vi "Trig Rate Charactarization.vi"(7 "Reset latch":refnum<vi>, 8 "error in (no error)":errorcluster, 9 "Programmatic set Vtrig":refnum<vi>, 11 "VTrig mV":refnum<vi>) -> (0 "Error out":errorcluster)   [LabVIEW 2016]
uses:
  <vilib>/Platform/TimedLoop/XDataNode/timing_clust.ctl
  <vilib>/Platform/TimedLoop/XDataNode/nitl_modes.ctl
  <vilib>/Platform/TimedLoop/XDataNode/wakeup.ctl
  <vilib>/platform/TimedLoop/XDataNode/XDataNode.xnode
  <vilib>/Platform/TimedLoop/XDataNode/XDNodeRunTimeDep.lvlib
  <vilib>/Analysis/NI_AALBase.lvlib
panel:
  out "Previous trigger level":dbl
  out "Trigger level increment":dbl
  out "Datapoints":i32
  out "Level number":i32
  out "Current\n trigger level":dbl
  in  "Datapoints per level":i32
  in  "finish level":bool
  in  "Bias being autoset?":bool=TRUE
  in  "MPPC Overvoltage":dbl
  in  "ROB ID":i32
  in  "MPPC Serial number":i32
  in  "Scintillator ID":i32
  in  "Data":i32[](array[numeric])
  out "Command Queue":string[](array[string])
  in  "stop":bool
  out "Hitrate histogram":T1(graph)
  out "Waveform Chart":dbl(graph)
  in  "Datasave path":path=path "D:/Data/Characterizations/Trigger rate characterizations"
  in  "Levels":i32
  in  "Range min":i32 format="%.0f  mV"
  in  "Range max":i32 format="%.0f mV"
  in  "Begin characterization":bool
  in  "Period":i32=1000 format="%.0f ms"
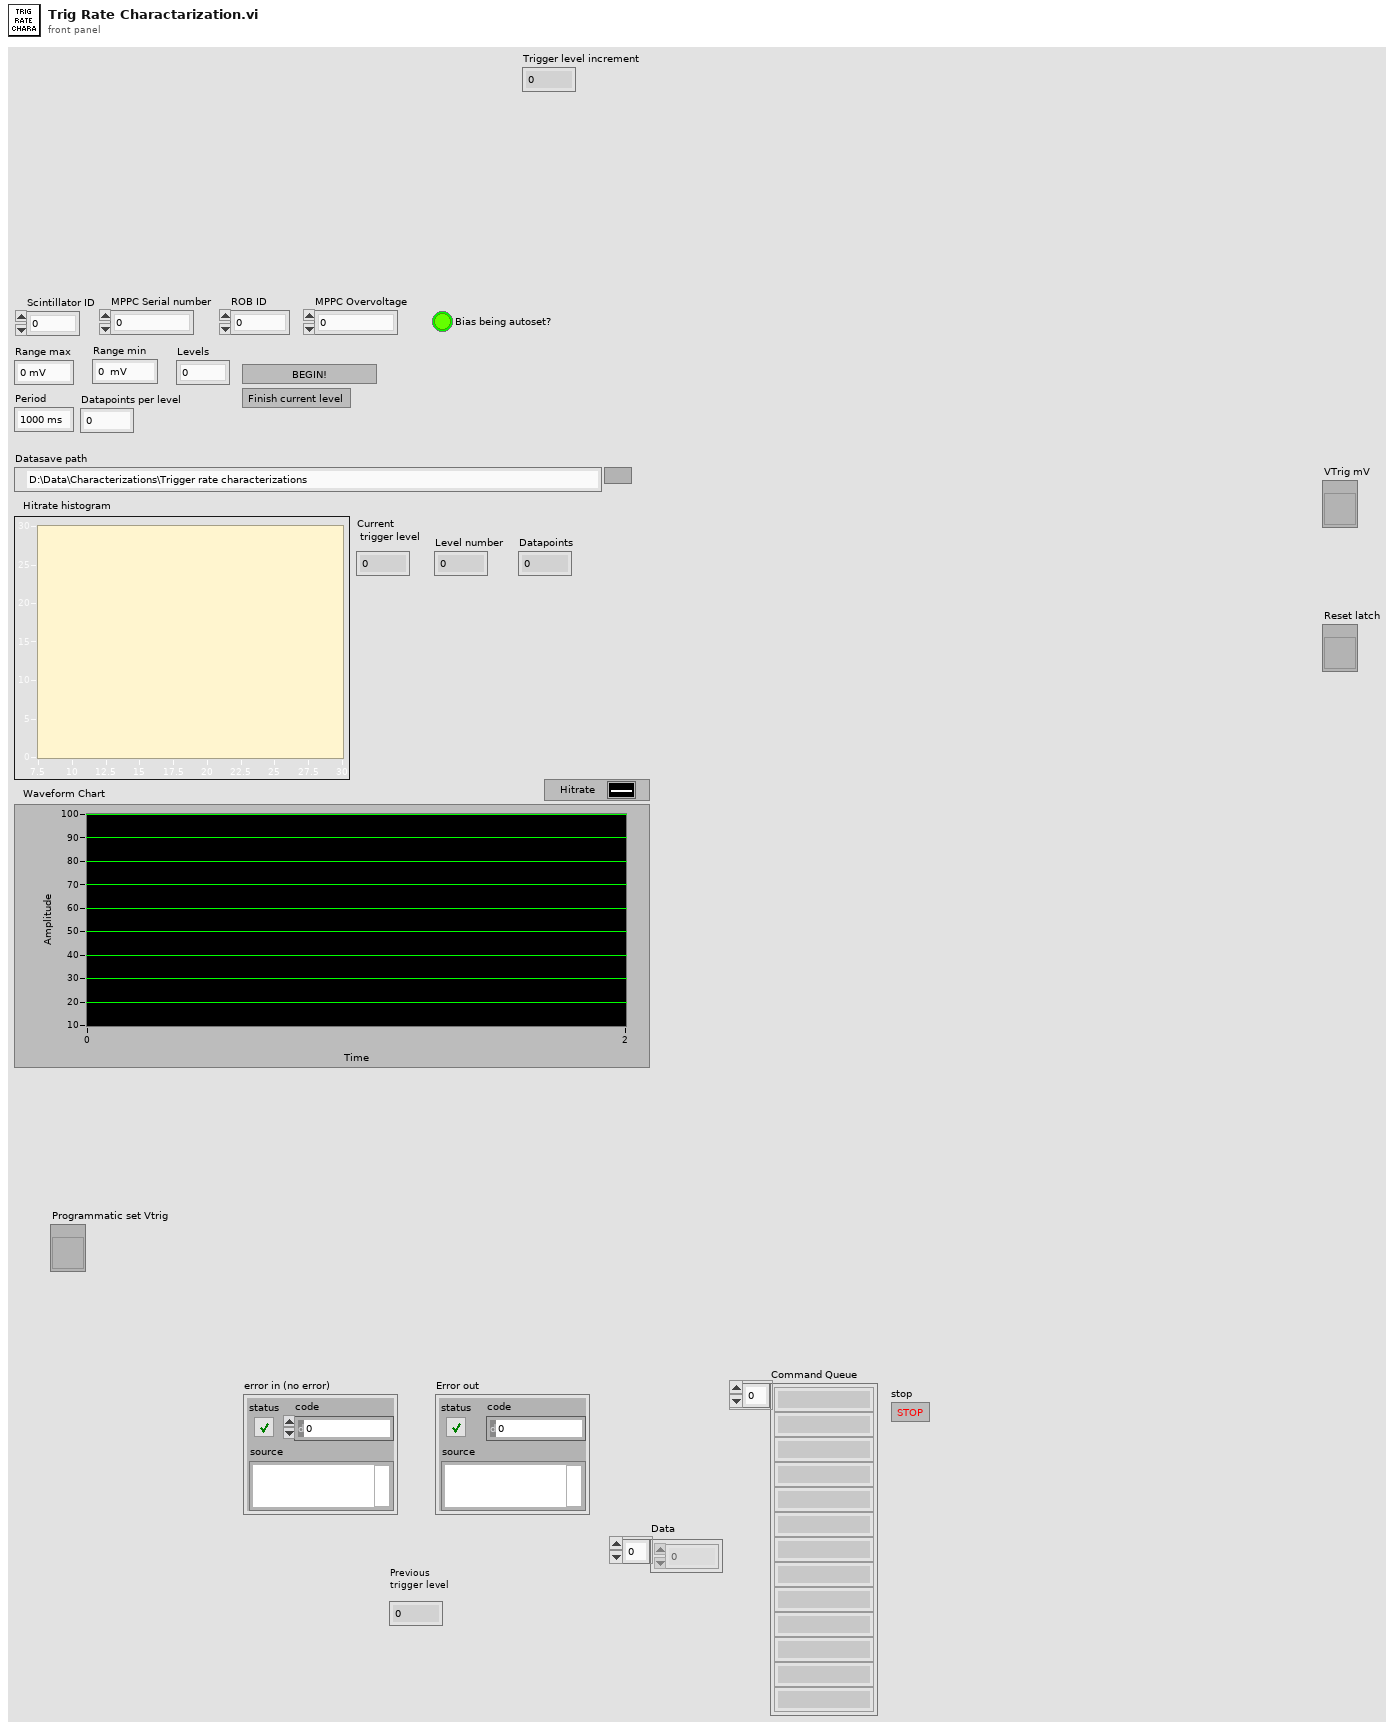
[diagram p1: front panel]
types:
  T1 = cluster{"X Values":dbl[], "Histogram: h(x)":i32[]}
  T2 = enum16{"open", "replace", "create", "open or create", "replace or create", "replace or create with confirmation"}
  T3 = enum16{"Reset", "ReadAndReset", "Read", "Add", "Init"}
  T4 = typedef "XDNodeRunTimeDep.lvlib/timing_clust.ctl" = cluster{"Expected End [f-1]":u64, "Actual End [f-1]":u64, "Finished Late? [f-1]":bool, "Expected End [i-1]":u64, "Actual End [i-1]":u64, "Finished Late? [i-1]":bool, "Expected Start [i]":u64, "Actual Start [i]":u64, "Expected Start [f]":u64, "Actual Start [f]":u64, "Source Name":string, "Structure Name":string, "Period":i64, "Deadline":i64, "Offset":i64, "Start":i64, "Priority":i32, "Timeout":i32, "Mode":T5, "Wakeup Reason":T6, "Error":errorcluster, "Source Type":string, "Secondary Source Type":string, "Global End Time":u64, "Global Start Time":u64, "Frame Duration":u64, "Iteration Duration":u64, "Assigned CPU":i32, "I/O Scan Engine Mode":u32}
  T5 = typedef "XDNodeRunTimeDep.lvlib/nitl_modes.ctl" = enum32{"No Change", "Process missed periods, maintain original phase", "Discard missed periods, maintain original phase", "Process missed periods, ignore original phase", "Discard missed periods, ignore original phase"}
  T6 = typedef "XDNodeRunTimeDep.lvlib/wakeup.ctl" = enum32{"Normal", "Aborted", "Asynchronous wakeup", "Timing source error", "Timed loop error", "Timeout"}
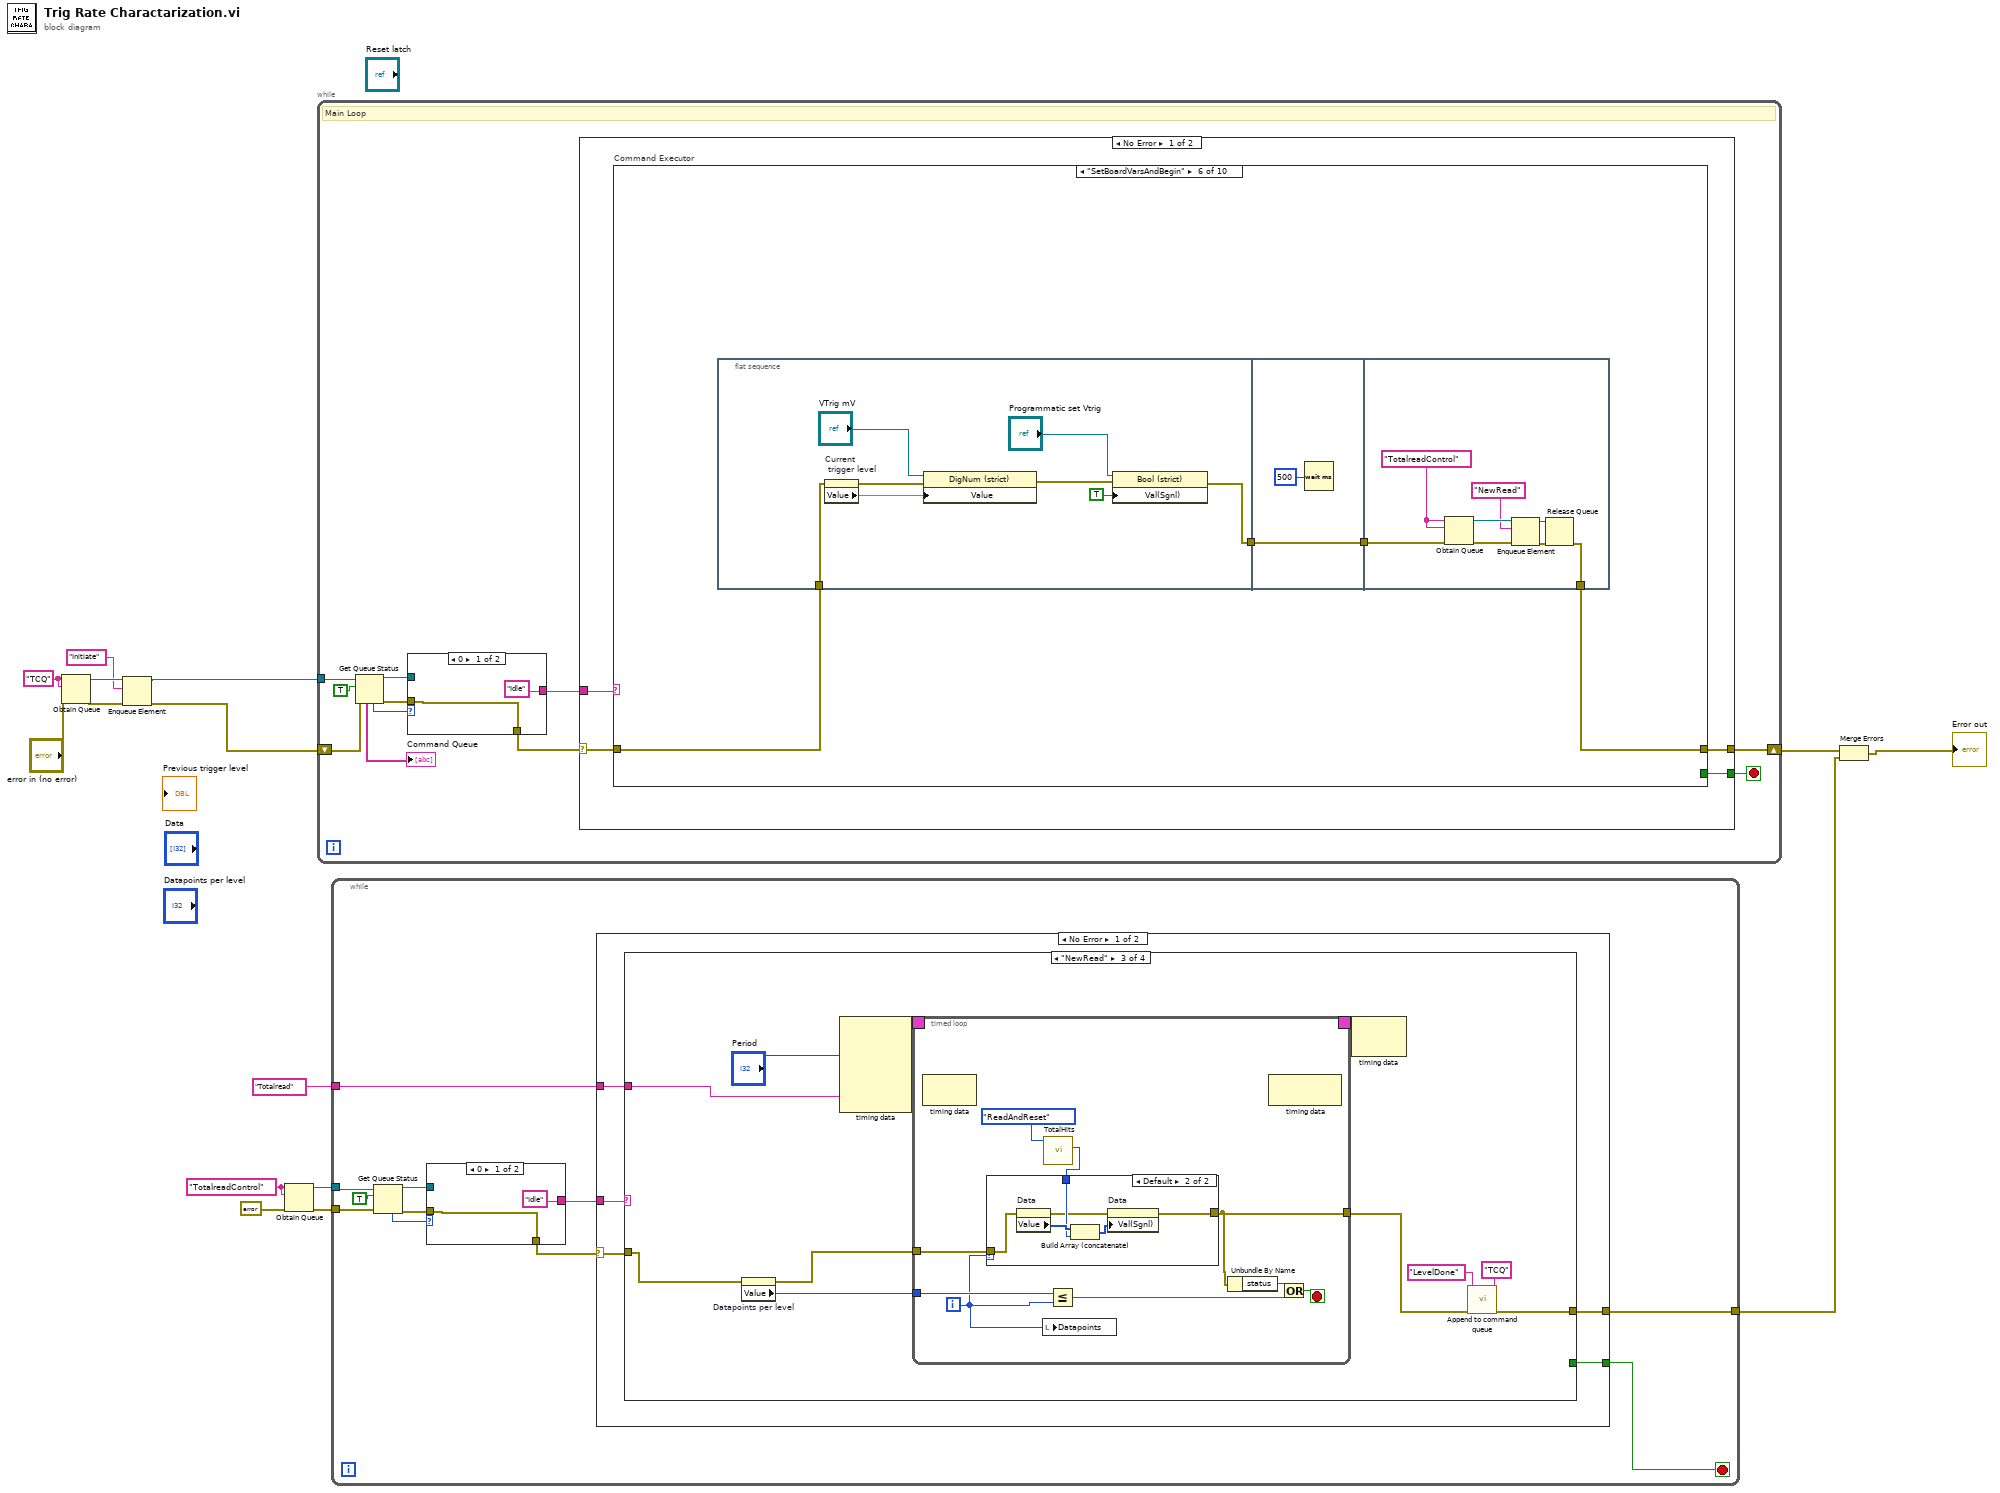
[diagram p0: block diagram]
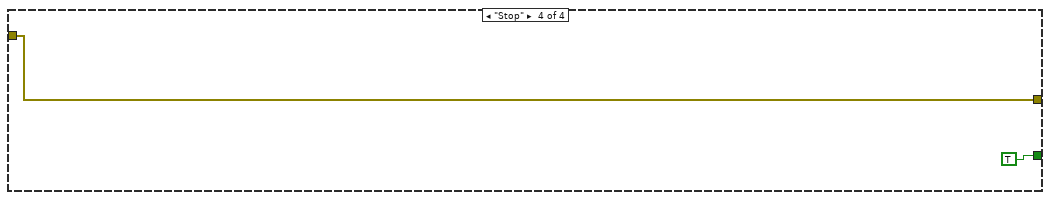
[diagram p5: hidden frame]
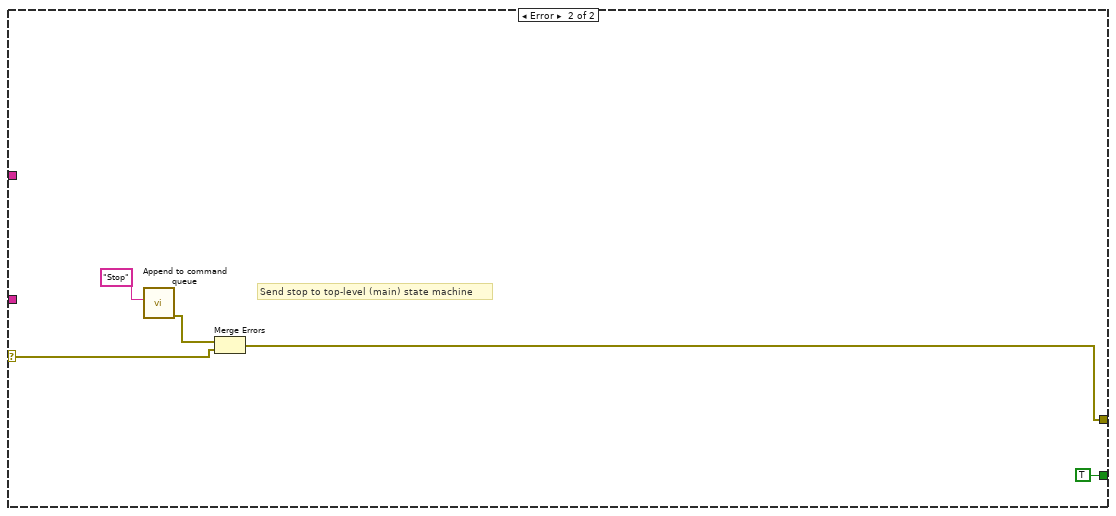
[diagram p6: hidden frame]
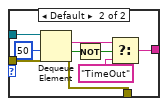
[diagram p7: hidden frame]
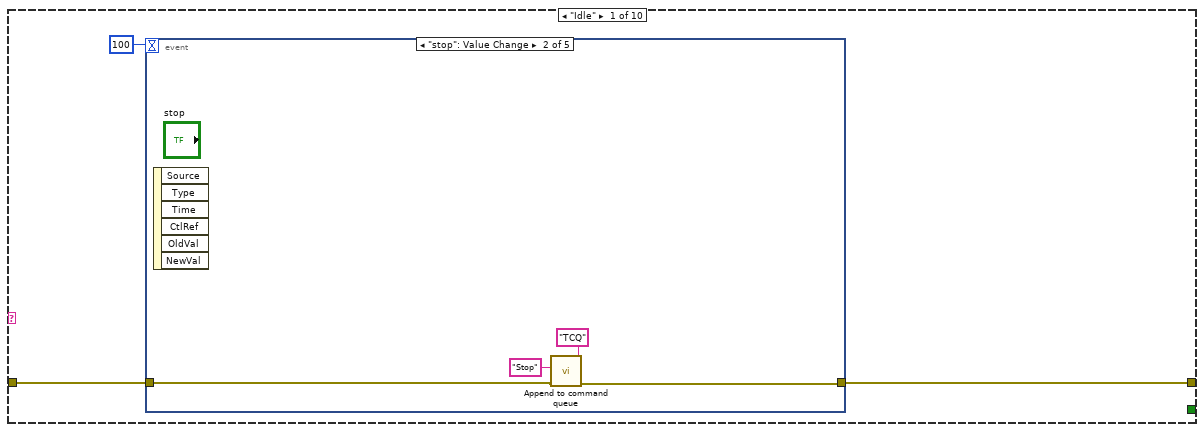
[diagram p8: hidden frame]
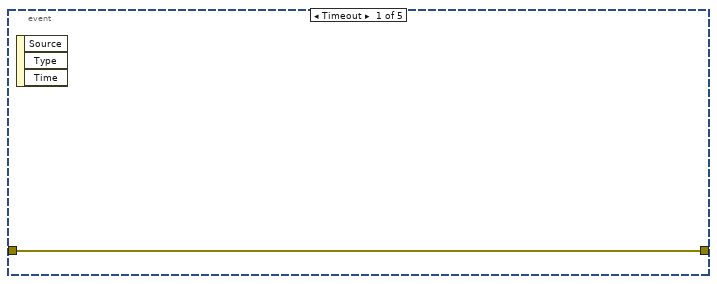
[diagram p9: hidden frame]
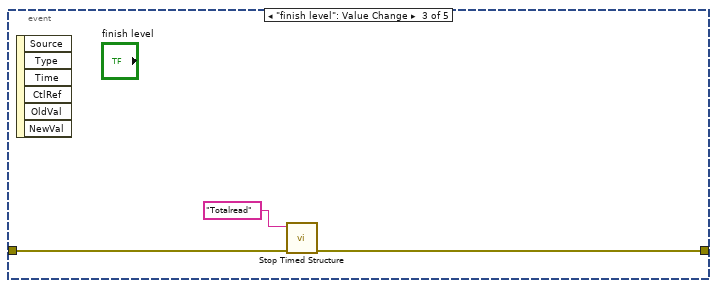
[diagram p10: hidden frame]
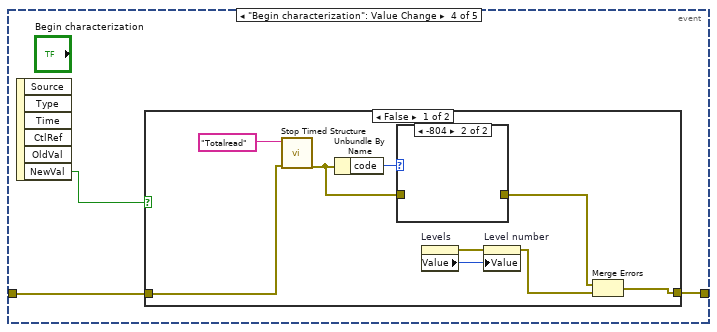
[diagram p11: hidden frame]
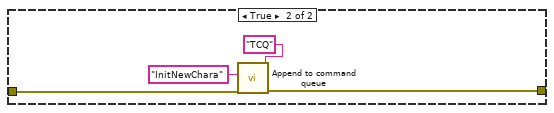
[diagram p13: hidden frame]
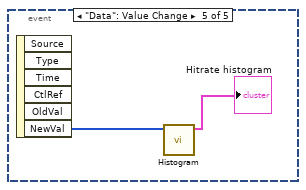
[diagram p14: hidden frame]
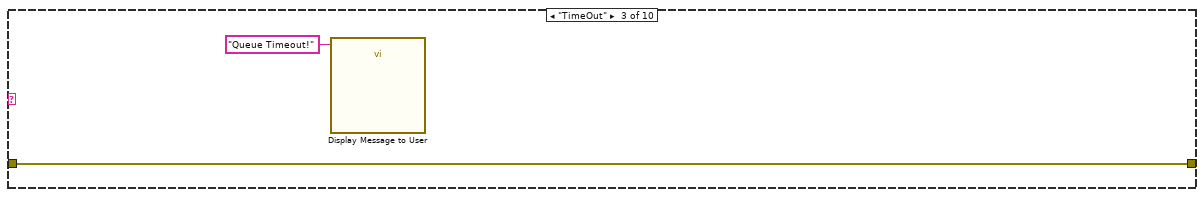
[diagram p16: hidden frame]
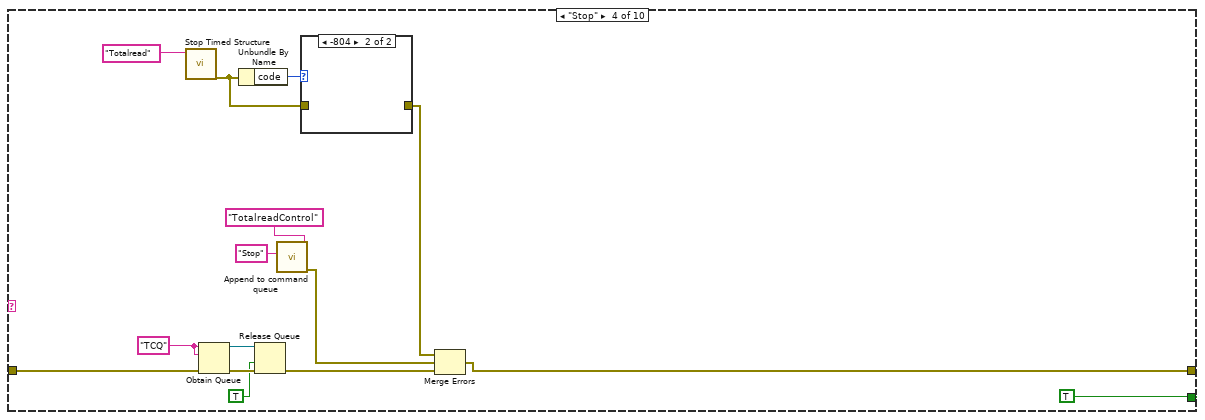
[diagram p17: hidden frame]
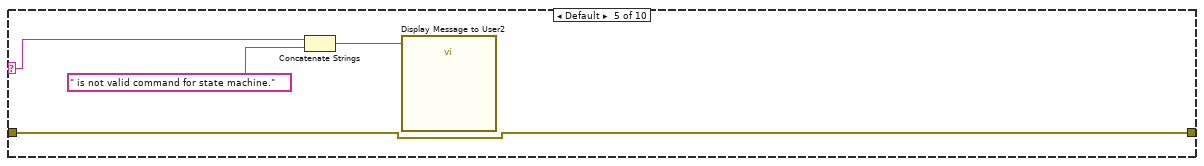
[diagram p19: hidden frame]
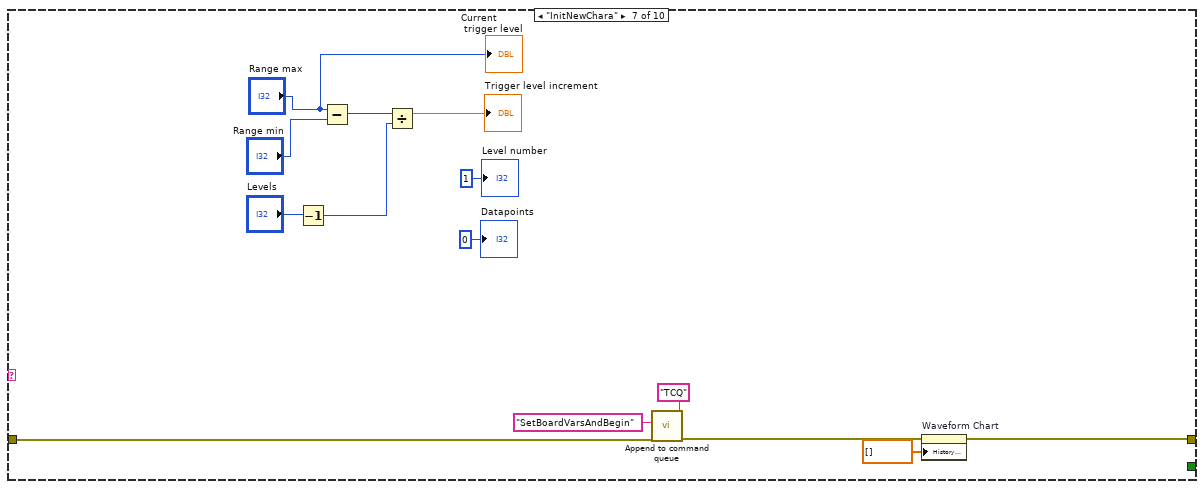
[diagram p20: hidden frame]
diagram:
  w7 = "TotalreadControl" ("name (unnamed)")
  w15 = "TCQ" ("name (unnamed)")
  n1 = Obtain Queue(name (unnamed)=w15, element data type=w15, error in (no error)="error in (no error)") -> (queue out=w13:refnum<queue>, error out=w11:errorcluster)  [unwired: 2 in, 1 out]
  n2 = Enqueue Element(queue=w13, element="Initiate", error in (no error)=w11) -> (queue out=w4:refnum<queue>, error out=w10:errorcluster)  [unwired: 1 in, 1 out]
  n3 = Obtain Queue(name (unnamed)=w7, element data type=w7, error in (no error)=errorcluster {"status"=FALSE, "code"=0, "source"=""}) -> (queue out=w6:refnum<queue>, error out=w5:errorcluster)  [unwired: 2 in, 1 out]
  n4 = while {
    tunnel: w4 -> [w22]
    shift-right: [w18] -> w3
    shift-left: w10 -> [w19]
    stop <- w17 stop-if-true
    # "Main Loop"
    n5 = Get Queue Status(queue=w22, return elements? (F)=TRUE, error in (no error)=w19) -> (queue out=w25:refnum<queue>, error out=w24:errorcluster, # elements in queue=w26:i32, elements=→"Command Queue":string[])  [unwired: 4 out]
    n6 = case shown="0" w26 {
      tunnel: ["Idle" ("element") w256] -> w20
      tunnel: w25 -> [_ w262]
      tunnel: w24 -> [w252 w261]
      tunnel: [w252 w255] -> w16
      frame 0 {
      }
      frame Default {
        n7 = Dequeue Element(queue=w262, timeout in ms (-1)=50, error in (no error)=w261) -> (element=w260:string, timed out?=w259:bool, error out=w255:errorcluster)  [unwired: 1 out]
        n8 = Not(x=w259) -> (.not. x?=w258:bool)
        n9 = Select(t=w260, s=w258, f="TimeOut") -> (s? t:f=w256:string)
      }
    }
    n10 = case shown="No Error" w16 {
      selector: w16 -> [w27 w244]
      tunnel: w20 -> [w30 _]
      tunnel: [w29 w243] -> w18
      tunnel: [w28 TRUE] -> w17
      frame No Error {
        n11 = case "Command Executor" shown="\"SetBoardVarsAndBegin\"" w30 {
          selector: w30 -> [_ _ _ _ w81 _ _ _ _ _]
          tunnel: [w31 w61 w62 w64 w80 w84 w107 w127 w164 w229] -> w29
          tunnel: w27 -> [w32 w61 w62 w73 w80 w87 w112 w129 w166 w231]
          tunnel: [_ _ _ TRUE _ _ _ _ _ _] -> w28
          frame "Idle" {
            n12 = event shown="[1] \"stop\": Value Change" {
              selector: _ -> [_ _ _ _ _]
              dyn-events: _ -> [_ _ _ _ _]
              timeout: 100 -> [_ _ _ _ _]
              tunnel: w32 -> [w34 w38 w41 w44 _]
              tunnel: [w34 w37 w40 w43 _] -> w31
              event Timeout {
                n13 = event-data() -> ()  [unwired: 1 in, 3 out]
              }
              event "stop": Value Change {
                n14 = event-data() -> ()  [unwired: 1 in, 6 out]
                n15 = call "Append to command queue.vi"("Name (CommandQueue)"="TCQ", "error in (no error)"=w38, "Single command"="Stop") -> ("error out"=w37:errorcluster)  [unwired: 8 in]
              }
              event "finish level": Value Change {
                n16 = event-data() -> ()  [unwired: 1 in, 6 out]
                n17 = call <vilib>:"Stop Timed Structure.vi"("error in (no error)"=w41, "name"="Totalread" ("Structure Name")) -> ("error out"=w40:errorcluster)  [unwired: 9 in]
              }
              event "Begin characterization": Value Change {
                n18 = event-data() -> ("NewVal"=w42:bool)  [unwired: 1 in, 5 out]
                n19 = case shown="False" w42 {
                  tunnel: w44 -> [w48 w57]
                  tunnel: [w46 w56] -> w43
                  frame False {
                    n20 = call <vilib>:"Stop Timed Structure.vi"("error in (no error)"=w48, "name"="Totalread" ("Structure Name")) -> ("error out"=w49:errorcluster)  [unwired: 9 in]
                    n21 = Unbundle By Name(w49) -> ("code"=w50:i32)
                    n22 = case shown="-804" w50 {
                      tunnel: w49 -> [w54 _]
                      tunnel: [w54 _] -> w45
                      frame Default {
                      }
                      frame -804 {
                      }
                    }
                    n23 = property on="Levels" class="DigNum (strict)"() -> (error out=w52:errorcluster, "Value"=w53:i32)  [unwired: 2 in, 1 out]
                    n24 = property on="Level number" class="DigNum (strict)"(error in=w52, "Value"=w53) -> (error out=w47:errorcluster)  [unwired: 1 in, 1 out]
                    n25 = Merge Errors(w45, w47) -> (w46:errorcluster)
                  }
                  frame True {
                    n26 = call "Append to command queue.vi"("Name (CommandQueue)"="TCQ", "error in (no error)"=w57, "Single command"="InitNewChara") -> ("error out"=w56:errorcluster)  [unwired: 8 in]
                  }
                }
              }
              event "Data": Value Change {
                n27 = event-data() -> ("NewVal"=w59:i32[])  [unwired: 1 in, 5 out]
                n28 = call <vilib>:"Histogram.vi"("X"=w59) -> ("Histogram Graph"=→"Hitrate histogram":T1)  [unwired: 7 in, 3 out]
              }
            }
          }
          frame "Initiate" {
          }
          frame "TimeOut" {
            n29 = call "Display Message to User"("Message"="Queue Timeout!" ("string")) -> ()  [unwired: 9 in, 2 out]
          }
          frame "Stop" {
            w74 = "TCQ" ("name (unnamed)")
            n30 = call <vilib>:"Stop Timed Structure.vi"("name"="Totalread" ("Structure Name")) -> ("error out"=w66:errorcluster)  [unwired: 10 in]
            n31 = Obtain Queue(name (unnamed)=w74, element data type=w74, error in (no error)=w73) -> (queue out=w77:refnum<queue>, error out=w76:errorcluster)  [unwired: 2 in, 1 out]
            n32 = Unbundle By Name(w66) -> ("code"=w69:i32)
            n33 = Release Queue(queue=w77, force destroy? (F)=TRUE, error in (no error)=w76) -> (error out=w67:errorcluster)  [unwired: 2 out]
            n34 = call "Append to command queue.vi"("Name (CommandQueue)"="TotalreadControl", "Single command"="Stop") -> ("error out"=w68:errorcluster)  [unwired: 9 in]
            n35 = case shown="-804" w69 {
              tunnel: w66 -> [w79 _]
              tunnel: [w79 _] -> w65
              frame Default {
              }
              frame -804 {
              }
            }
            n36 = Merge Errors(w65, w68, w67) -> (w64:errorcluster)
          }
          frame Default {
            n37 = Concatenate Strings(w81, " is not valid command for state machine." ("string")) -> (w82:string)
            n38 = call "Display Message to User2"("Message"=w82) -> ()  [unwired: 9 in, 2 out]
          }
          frame "SetBoardVarsAndBegin" {
            n39 = flat-sequence {
              tunnel: w87 -> [w90]
              tunnel: [w89] -> w86
              tunnel: w86 -> [w96]
              tunnel: [w96] -> w85
              tunnel: w85 -> [w100]
              tunnel: [w99] -> w84
              frame #0 {
                n40 = property on="Current\n trigger level" class="DigNum (strict)"(error in=w90) -> (error out=w92:errorcluster, "Value"=w93:dbl)  [unwired: 1 in, 1 out]
                n41 = property class="DigNum (strict)"(reference="VTrig mV", error in=w92, "Value"=w93) -> (error out=w91:errorcluster)  [unwired: 1 out]
                n42 = property class="Bool (strict)"(reference="Programmatic set Vtrig", error in=w91, "Val(Sgnl)"=TRUE ("Value (Signaling)")) -> (error out=w89:errorcluster)  [unwired: 1 out]
              }
              frame #1 {
                n43 = Wait (ms)(milliseconds to wait=u32 500) -> ()  [unwired: 1 out]
              }
              frame #2 {
                w101 = "TotalreadControl" ("name (unnamed)")
                n44 = Obtain Queue(name (unnamed)=w101, element data type=w101, error in (no error)=w100) -> (queue out=w105:refnum<queue>, error out=w104:errorcluster)  [unwired: 2 in, 1 out]
                n45 = Enqueue Element(queue=w105, element="NewRead", error in (no error)=w104) -> (queue out=w102:refnum<queue>, error out=w103:errorcluster)  [unwired: 1 in, 1 out]
                n46 = Release Queue(queue=w102, error in (no error)=w103) -> (error out=w99:errorcluster)  [unwired: 1 in, 2 out]
              }
            }
          }
          frame "InitNewChara" {
            n47 = Decrement(x="Levels") -> (x-1=w109:i32)
            n48 = Subtract(x="Range max", y="Range min") -> (x-y=w117:i32)
            n49 = Divide(x=w117, y=w109) -> (x/y=→"Trigger level increment":dbl)
            n50 = call "Append to command queue.vi"("Name (CommandQueue)"="TCQ", "error in (no error)"=w112, "Single command"="SetBoardVarsAndBegin") -> ("error out"=w108:errorcluster)  [unwired: 8 in]
            n51 = property on="Waveform Chart" class="WFChart (strict)"(error in=w108, "History Data"=dbl[] []) -> (error out=w107:errorcluster)  [unwired: 1 in, 1 out]
            "Current\n trigger level" <- "Range max"
            "Level number" <- 1 ("Level number")
            "Datapoints" <- 0 ("Datapoints")
          }
          frame "LevelDone" {
            n52 = property on="Levels" class="DigNum (strict)"(error in=w129) -> (error out=w130:errorcluster, "Value"=w131:i32)  [unwired: 1 in, 1 out]
            n53 = property on="Level number" class="DigNum (strict)"(error in=w130) -> (error out=w124:errorcluster, "Value"=w132:i32)  [unwired: 1 in, 1 out]
            n54 = Equal?(x=w132, y=w131) -> (x = y?=w128:bool)
            n55 = call "Append to command queue.vi"("Name (CommandQueue)"="TCQ", "error in (no error)"=w124, "Single command"="SaveData") -> ("error out"=w121:errorcluster)  [unwired: 8 in]
            n56 = property on="Current\n trigger level" class="DigNum (strict)"(error in=w121) -> (error out=w122:errorcluster, "Value"=w123:dbl)  [unwired: 1 in, 1 out]
            n57 = property on="Previous trigger level" class="DigNum (strict)"(error in=w122, "Value"=w123) -> (error out=w120:errorcluster)  [unwired: 1 in, 1 out]
            n58 = case shown="False" w128 {
              tunnel: w120 -> [w138 w149]
              tunnel: [w135 w148] -> w127
              frame False {
                n59 = property on="Trigger level increment" class="DigNum (strict)"(error in=w138) -> (error out=w143:errorcluster, "Value"=w142:dbl)  [unwired: 1 in, 1 out]
                n60 = property on="Current\n trigger level" class="DigNum (strict)"(error in=w143) -> (error out=w140:errorcluster, "Value"=w133:dbl)  [unwired: 1 in, 1 out]
                n61 = Subtract(x=w133, y=w142) -> (x-y=w141:dbl)
                n62 = property on="Current\n trigger level" class="DigNum (strict)"(error in=w140, "Value"=w141) -> (error out=w139:errorcluster)  [unwired: 1 in, 1 out]
                n63 = property on="Level number" class="DigNum (strict)"(error in=w139) -> (error out=w144:errorcluster, "Value"=w146:i32)  [unwired: 1 in, 1 out]
                n64 = Increment(x=w146) -> (x+1=w145:i32)
                n65 = property on="Level number" class="DigNum (strict)"(error in=w144, "Value"=w145) -> (error out=w134:errorcluster)  [unwired: 1 in, 1 out]
                n66 = call "Append to command queue.vi"("Name (CommandQueue)"="TCQ", "error in (no error)"=w134, "Single command"="SetBoardVarsAndBegin") -> ("error out"=w135:errorcluster)  [unwired: 8 in]
              }
              frame True {
                n67 = call "Append to command queue.vi"("Name (CommandQueue)"="TCQ", "error in (no error)"=w149, "Single command"="Reset") -> ("error out"=w148:errorcluster)  [unwired: 8 in]
              }
            }
          }
          frame "SaveData" {
            w155 = "\t"
            n68 = control-ref of="Period"() -> (w205:refnum<vi>)
            n69 = control-ref of="Previous trigger level"() -> (w158:refnum<vi>)
            n70 = property class="DigNum (strict)"(reference=w205, error in=w166) -> (error out=w191:errorcluster, "Value"=w174:i32)  [unwired: 1 out]
            n71 = property class="DigNum (strict)"(reference=w158, error in=w191) -> (error out=w190:errorcluster, "Value"=w206:dbl)  [unwired: 1 out]
            n72 = property on="Data" class="Arr (strict)"(error in=w190) -> (error out=w189:errorcluster, "Value"=w173:i32[])  [unwired: 1 in, 1 out]
            n73 = property on="Datasave path" class="Path"(error in=w166) -> (error out=w165:errorcluster, "Value"=w187:path)  [unwired: 1 in, 1 out]
            n74 = Build Path(base path=w187, name or relative path="Summary.csv") -> (appended path=w182:path)
            n75 = Number To Decimal String(number=w206) -> (decimal integer string=w170:string)  [unwired: 1 in]
            n76 = Number To Decimal String(number=w174) -> (decimal integer string=w157:string)  [unwired: 1 in]
            n77 = Open/Create/Replace File(file path (use dialog)=w182, error in=w165, operation (0:open)=T2."open") -> (refnum out=w185:refnum<file>, error out=w184:errorcluster)  [unwired: 3 in, 1 out]
            n78 = Unbundle By Name(w184) -> ("code"=w183:i32)
            n79 = Concatenate Strings(w170, "mV " ("string"), w157, "s.csv " ("string")) -> (w204:string)
            n80 = Array To Spreadsheet String(delimiter (Tab)="\r\n", array=w173, 3:"%d" ("format string")) -> (spreadsheet string=w197:string)
            n81 = Build Path(base path="Datasave path", name or relative path=w204) -> (appended path=w209:path)
            n82 = call "Build header single level.vi"("Overvoltage"="MPPC Overvoltage", "Recommended at 25C"="Bias being autoset?", "MPPC Serial number"="MPPC Serial number", "ROB ID"="ROB ID", "Scintillator ID"="Scintillator ID") -> ("Header"=w181:string)  [unwired: 6 in]
            n83 = case shown="7" w183 {
              tunnel: w185 -> [_ w228]
              tunnel: w184 -> [_ w227]
              tunnel: w182 -> [w220 _]
              tunnel: w181 -> [w215 _]
              tunnel: [w217 w223] -> w175
              tunnel: [w216 w222] -> w176
              frame 7 {
                n84 = Open/Create/Replace File(file path (use dialog)=w220, operation (0:open)=T2."create") -> (refnum out=w218:refnum<file>, error out=w219:errorcluster)  [unwired: 4 in, 1 out]
                n85 = Concatenate Strings(w215, "Trigger\tmean\tstandard deviation\tvariance\tpool size\tperiod" ("delimiter (Tab)"), "\r\n") -> (w213:string)
                n86 = Write to Text File(file (use dialog)=w218, text=w213, error in=w219) -> (refnum out=w217:refnum<file>, error out=w216:errorcluster)  [unwired: 1 in, 1 out]
              }
              frame Default {
                n87 = Get File Size(file=w228, error in=w227) -> (refnum out=w226:refnum<file>, size (in bytes)=w225:i64, 0:w224:errorcluster)
                n88 = Set File Position(offset (in bytes) (0)=w225, refnum=w226, error in=w224) -> (refnum out=w223:refnum<file>, error out=w222:errorcluster)  [unwired: 1 in]
              }
            }
            n89 = Concatenate Strings(w181, w197) -> (w194:string)
            n90 = Open/Create/Replace File(file path (use dialog)=w209, error in=w189, operation (0:open)=T2."open or create") -> (refnum out=w196:refnum<file>, error out=w195:errorcluster)  [unwired: 3 in, 1 out]
            n91 = call <vilib>:"Std Deviation and Variance.vi"("X"=w173) -> ("mean"=w159:dbl, "standard deviation"=w180:dbl, "variance"=w179:dbl)  [unwired: 1 in]
            "Waveform Chart" <- w159
            n92 = Array Size(array=w173) -> (size(s)=w172:i32)
            n93 = Build Array(w159, w180, w179) -> (w177:dbl[])
            n94 = Number To Decimal String(number=w172) -> (decimal integer string=w169:string)  [unwired: 1 in]
            n95 = Write to Text File(file (use dialog)=w196, text=w194, error in=w195) -> (refnum out=w193:refnum<file>, error out=w192:errorcluster)  [unwired: 1 in, 1 out]
            n96 = Array To Spreadsheet String(array=w177, 3:"%5.3f" ("format string")) -> (spreadsheet string=w154:string)  [unwired: 1 in]
            n97 = Close File(refnum=w193, error in=w192) -> (error out=w162:errorcluster)  [unwired: 1 out]
            n98 = Search/Split String(string=w154, search string/char (-)="\r\n") -> (substring before match=w152:string)  [unwired: 1 in, 2 out]
            n99 = Concatenate Strings(w170, w155, w152, w155, w169, w155, w157, "\r\n") -> (w171:string)
            n100 = Write to Text File(file (use dialog)=w175, text=w171, error in=w176) -> (refnum out=w167:refnum<file>, error out=w168:errorcluster)  [unwired: 1 in, 1 out]
            n101 = property on="Data" class="Arr (strict)"(error in=w162, "Value"=i32[] [] ("Data")) -> (error out=w161:errorcluster)  [unwired: 1 in, 1 out]
            n102 = Close File(refnum=w167, error in=w168) -> (error out=w163:errorcluster)  [unwired: 1 out]
            n103 = Merge Errors(w163, w161) -> (w164:errorcluster)
          }
          frame "Reset" {
            n104 = property on="Level number" class="DigNum (strict)"(error in=w231, "Value"=1 ("Level number")) -> (error out=w230:errorcluster)  [unwired: 1 in, 1 out]
            n105 = property on="Datapoints" class="DigNum (strict)"(error in=w230, "Value"=0 ("Datapoints")) -> (error out=w229:errorcluster)  [unwired: 1 in, 1 out]
          }
        }
      }
      frame Error {
        w246 = "TCQ" ("name (unnamed)")
        n106 = call <vilib>:"Stop Timed Structure.vi"("name"="Totalread" ("Structure Name")) -> ("error out"=w235:errorcluster)  [unwired: 10 in]
        n107 = Obtain Queue(name (unnamed)=w246, element data type=w246) -> (queue out=w249:refnum<queue>, error out=w248:errorcluster)  [unwired: 3 in, 1 out]
        n108 = Unbundle By Name(w235) -> ("code"=w236:i32)
        n109 = call "Append to command queue.vi"("Single command"="Stop") -> ("error out"=w241:errorcluster)  [unwired: 10 in]
        n110 = Release Queue(queue=w249, force destroy? (F)=TRUE, error in (no error)=w248) -> (error out=w245:errorcluster)  [unwired: 2 out]
        n111 = case shown="-804" w236 {
          tunnel: w235 -> [w251 _]
          tunnel: [w251 _] -> w234
          frame Default {
          }
          frame -804 {
          }
        }
        n112 = call "Append to command queue.vi"("Name (CommandQueue)"="TotalreadControl", "Single command"="Stop") -> ("error out"=w238:errorcluster)  [unwired: 9 in]
        n113 = Merge Errors(w234, w238, w241, w245, w244) -> (w243:errorcluster)
      }
    }
  }
  n114 = while {
    tunnel: "Totalread" ("Structure Name") -> [w273]
    tunnel: w6 -> [w268]
    tunnel: w5 -> [w267]
    tunnel: [w264] -> w2
    stop <- w263 stop-if-true
    n115 = Get Queue Status(queue=w268, return elements? (F)=TRUE, error in (no error)=w267) -> (queue out=w271:refnum<queue>, error out=w270:errorcluster, # elements in queue=w272:i32)  [unwired: 5 out]
    n116 = case shown="0" w272 {
      tunnel: ["Idle" ("element") w326] -> w266
      tunnel: w271 -> [_ w332]
      tunnel: w270 -> [w322 w331]
      tunnel: [w322 w325] -> w265
      frame 0 {
      }
      frame Default {
        n117 = Dequeue Element(queue=w332, timeout in ms (-1)=50, error in (no error)=w331) -> (element=w330:string, timed out?=w329:bool, error out=w325:errorcluster)  [unwired: 1 out]
        n118 = Not(x=w329) -> (.not. x?=w328:bool)
        n119 = Select(t=w330, s=w328, f="TimeOut") -> (s? t:f=w326:string)
      }
    }
    n120 = case shown="No Error" w265 {
      selector: w265 -> [w276 w319]
      tunnel: w273 -> [w278 _]
      tunnel: w266 -> [w277 _]
      tunnel: [w275 w318] -> w264
      tunnel: [w274 TRUE] -> w263
      frame No Error {
        n121 = case shown="\"NewRead\"" w277 {
          tunnel: w278 -> [_ _ w291 _]
          tunnel: [w279 w280 w290 w316] -> w275
          tunnel: w276 -> [w279 w280 w289 w316]
          tunnel: [_ _ _ TRUE] -> w274
          frame "TimeOut" {
          }
          frame Default {
          }
          frame "NewRead" {
            n122 = property on="Datapoints per level" class="DigNum (strict)"(error in=w289) -> (error out=w282:errorcluster, "Value"=w281:i32)  [unwired: 1 in, 1 out]
            n123 = node-c288("Period", w291) -> (w288:T4)  [unwired: 3 in]
            n124 = timed-loop {
              timing: w288 -> [_]
              timing-out: [_] -> w287
              tunnel: w282 -> [w298]
              tunnel: [w296] -> w283
              tunnel: w281 -> [w297]
              i -> [w292]
              stop <- w293 stop-if-true
              n125 = node-c288() -> ()  [unwired: 1 in, 1 out]
              n126 = local write "Datapoints"(w292) -> ()
              n127 = call "TotalHits.vi"("Action"=T3."ReadAndReset") -> ("Result"=w299:u64)  [unwired: 10 in]
              n128 = case shown="Default" w292 {
                tunnel: w299 -> [_ w306]
                tunnel: w298 -> [w301 w303]
                tunnel: [w301 w302] -> w296
                frame 0 {
                }
                frame Default {
                  n129 = property on="Data" class="Arr (strict)"(error in=w303) -> (error out=w304:errorcluster, "Value"=w307:i32[])  [unwired: 1 in, 1 out]
                  n130 = Build Array (concatenate)(w307, w306) -> (w305:u64[])
                  n131 = property on="Data" class="Arr (strict)"(error in=w304, "Val(Sgnl)"=w305) -> (error out=w302:errorcluster)  [unwired: 1 in, 1 out]
                }
              }
              n132 = Less Or Equal?(x=w297, y=w292) -> (x <= y?=w294:bool)
              n133 = Unbundle By Name(w296) -> ("status"=w295:bool)
              n134 = node-c288() -> ()  [unwired: 1 in, 1 out]
              n135 = Or(x=w295, y=w294) -> (x .or. y?=w293:bool)
            }
            n136 = node-c288(w287) -> ()  [unwired: 1 out]
            n137 = call "Append to command queue.vi"("Name (CommandQueue)"="TCQ" ("name (unnamed)"), "error in (no error)"=w283, "Single command"="LevelDone") -> ("error out"=w290:errorcluster)  [unwired: 8 in]
          }
          frame "Stop" {
          }
        }
      }
      frame Error {
        # "Send stop to top-level (main) state machine"
        n138 = call "Append to command queue.vi"("Single command"="Stop") -> ("error out"=w320:errorcluster)  [unwired: 10 in]
        n139 = Merge Errors(w320, w319) -> (w318:errorcluster)
      }
    }
  }
  n140 = Merge Errors(w3, w2) -> (→"Error out":errorcluster)
